vi "Write I16 Value.vi"(8 "error in (no error)":errorcluster, 10 "I16":i16, 11 "Numeric in":refnum<class "Abs_Single Float.lvclass">) -> (0 "error out":errorcluster, 3 "Numeric out":refnum<class "Abs_Single Float.lvclass">)   [LabVIEW 2021, in "Abs_Single Float.lvclass"]
uses:
  Abs_Single Float.lvclass
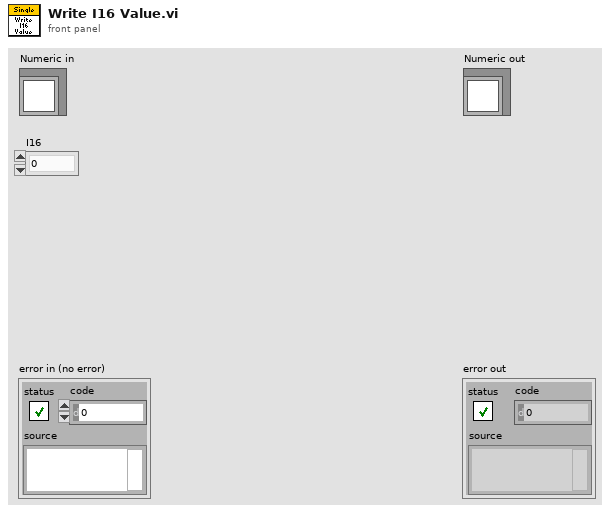
[diagram p1: front panel]
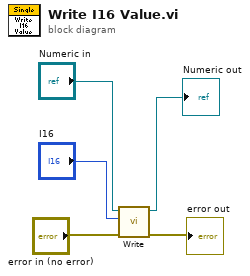
[diagram p0: block diagram]
diagram:
  n1 = call-dynamic "Write.vi"("error in (no error)"="error in (no error)", "Value"="I16", "Double Float.lvclass_340760 in"="Numeric in") -> ("error out"=→"error out":errorcluster, "Double Float.lvclass_340760 out"=→"Numeric out":refnum<class "Abs_Single Float.lvclass">)  [unwired: 7 in]
